vi "Lookup Node (ID).vi"(8 "error in (no error)":errorcluster, 10 "Node ID":u32, 11 "Cluster in":refnum<class "Cluster.lvclass">) -> (0 "error out":errorcluster, 2 "Node":refnum<class "Node.lvclass">, 3 "Cluster out":refnum<class "Cluster.lvclass">)   [LabVIEW 2020, in "VolatusConfig.lvlib" / "Cluster.lvclass"]
uses:
  Cluster.lvclass
  C:/dev/lv20CE/relink/lv-volatus/VolatusConfig/VolatusConfigElement/VolatusConfigElement.lvclass
  Node/Node.lvclass
  VolatusConfigElement/VolatusConfigElement.lvclass/VolatusConfigElement.ctl
  VolatusConfigElement/Element.vi
  lv-cdm/CDM-Config/Config Element/Lookup Descendants.vi
  lv-cdm/CDM-Config/Config Lookup/Match Meta.vi
  lv-cdm/CDM-Config/Config Element/Owner.vi
  lv-cdm/CDM-Config/Config Manager/Lookup Descendant.vi
  lv-cdm/CDM-Config/Config Element/Name.vi
  lv-cdm/CDM-Config/Config Filter/Config Lookup.lvclass
  Cluster.lvclass/Cluster.ctl
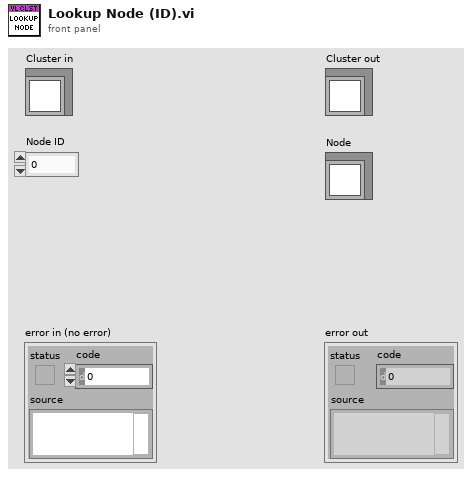
[diagram p1: front panel]
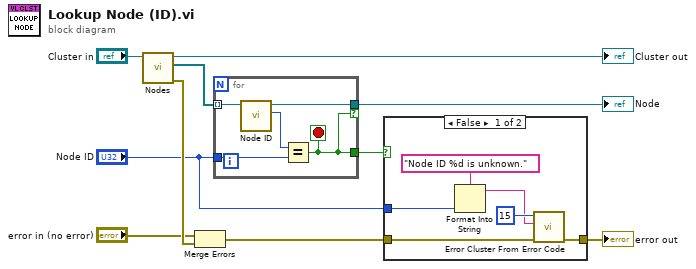
[diagram p0: block diagram]
diagram:
  n1 = call "Nodes.vi"("Cluster in"="Cluster in") -> ("error out"=w10:errorcluster, "Nodes"=w7:refnum<class "Node.lvclass">[], "Cluster out"=→"Cluster out":refnum<class "Cluster.lvclass">)  [unwired: 8 in]
  n2 = Merge Errors("error in (no error)", w10) -> (w3:errorcluster)
  n3 = for {
    tunnel: w7 -> [w15] mode=indexing
    tunnel: "Node ID" -> [w14]
    tunnel: [w12] -> w6 if=w11
    tunnel: [w11] -> w4
    stop <- w11 stop-if-true
    n4 = call "Node ID.vi"("Node in"=w15) -> ("Node ID"=w13:u32, "Node out"=w12:refnum<class "Node.lvclass">)  [unwired: 8 in, 1 out]
    n5 = Equal?(x=w13, y=w14) -> (x = y?=w11:bool)
  }
  "Node" <- w6
  n6 = case shown="False" w4 {
    tunnel: w3 -> [w21 w22]
    tunnel: [w20 w22] -> w2
    tunnel: "Node ID" -> [w16 _]
    frame False {
      n7 = Format Into String(format string="Node ID %d is unknown.", w16) -> (resulting string=w17:string)  [unwired: 2 in, 1 out]
      n8 = call <vilib>:"Error Cluster From Error Code.vi"("error in (no error)"=w21, "error message (\"\")"=w17, "error code (0)"=15) -> ("error out"=w20:errorcluster)  [unwired: 6 in]
    }
    frame True {
    }
  }
  "error out" <- w2
